vi "List Compatible Ctls.vi"(11 "UIP In":refnum<class "SizeUIP.lvclass">) -> (2 "Compatible Ctls":string[](array[string]), 3 "UIP Out":refnum<class "SizeUIP.lvclass">)   [LabVIEW 2015, in "SizeUIP.lvclass"]
doc: "Overwrite this method in your child UIPs to provide a custom list of vi server control classes compatible with that UIP."
uses:
  SizeUIP.lvclass
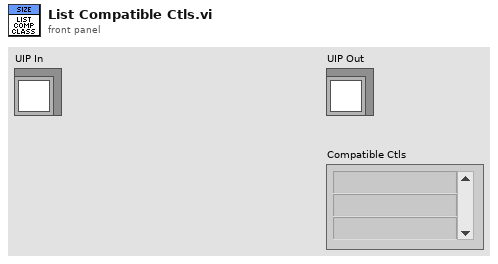
[diagram p1: front panel]
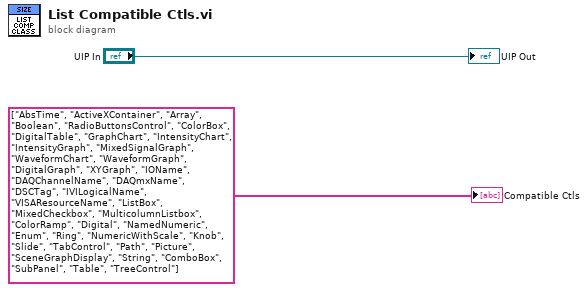
[diagram p0: block diagram]
diagram:
  "Compatible Ctls" <- string[] ["AbsTime", "ActiveXContainer", "Array", "Boolean", "RadioButtonsControl", "ColorBox", "DigitalTable", "GraphChart", "IntensityChart", "IntensityGraph", "MixedSignalGraph", "WaveformChart", "WaveformGraph", "DigitalGraph", "XYGraph", "IOName", "DAQChannelName", "DAQmxName", "DSCTag", "IVILogicalName", "VISAResourceName", "ListBox", "MixedCheckbox", "MulticolumnListbox", "ColorRamp", "Digital", "NamedNumeric", "Enum", "Ring", "NumericWithScale", "Knob", "Slide", "TabControl", "Path", "Picture", "SceneGraphDisplay", "String", "ComboBox", "SubPanel", "Table", "TreeControl"]
  "UIP Out" <- "UIP In"
